vi "Save Recall Setup.vi"(8 "error in (no error)":errorcluster, 9 "Address (1)":u32=1 min=1 max=5, 10 "Mode(F: Save)":bool, 11 "VISA resource name":refnum<visa-resource-name>) -> (0 "error out":errorcluster, 3 "VISA resource name out":refnum<visa-resource-name>)   [LabVIEW 2012, in "Agilent E364X Series.lvlib"]
doc: "This VI controls the memory functions of the DC power supply. The current system setup can be stored in one of five states (one of four states for the 668x series). These parameters are stored in memory locations 1 - 5."
uses:
  Agilent E364X Series.lvlib
panel:
  # "Recall"
  # "Save"
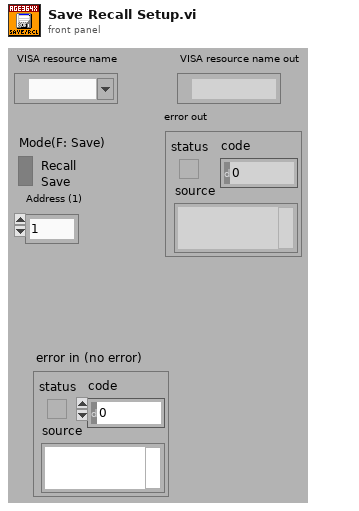
[diagram p1: front panel]
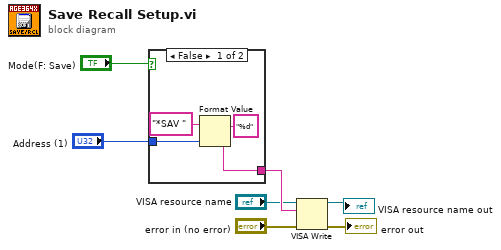
[diagram p0: block diagram]
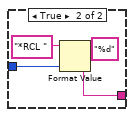
[diagram p2: hidden frame]
diagram:
  n1 = case shown="False" "Mode(F: Save)" {
    tunnel: [w11 w15] -> w6
    tunnel: "Address (1)" -> [w8 w12]
    frame False {
      n2 = Format Value(string ("")="*SAV ", format string="%d", value (0)=w8) -> (output string=w11:string)
    }
    frame True {
      n3 = Format Value(string ("")="*RCL ", format string="%d", value (0)=w12) -> (output string=w15:string)
    }
  }
  n4 = VISA Write(VISA resource name="VISA resource name", write buffer=w6, error in (no error)="error in (no error)") -> (VISA resource name out=→"VISA resource name out":refnum<visa-resource-name>, error out=→"error out":errorcluster)  [unwired: 1 out]
